vi "go_one_step.vi"(4 "执行完毕":bool, 5 "error in":errorcluster, 6 "Step":i32, 7 "Motor":i32, 8 "CmdLib In":refnum<k24>) -> (0 "error out":errorcluster, 1 "Position":i32, 2 "CmdLib Out":refnum<k24>)   [LabVIEW 2018]
uses:
  CmdLib.dll
  Verbal.vi
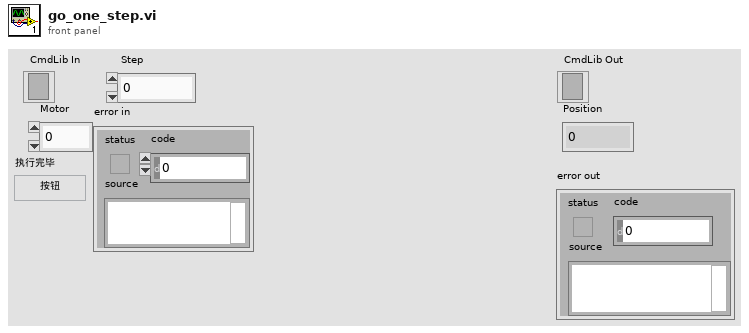
[diagram p1: front panel]
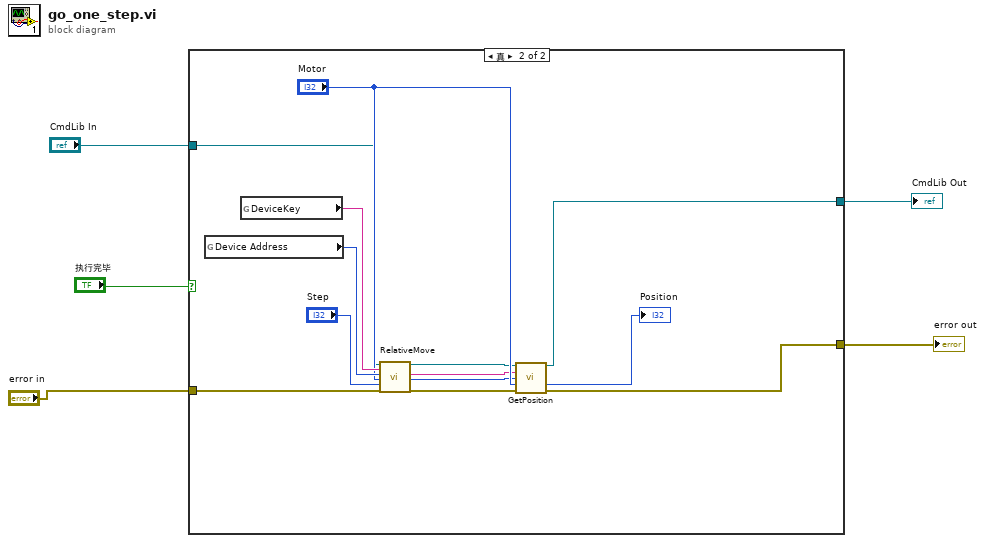
[diagram p0: block diagram]
diagram:
  n1 = case shown="真" "执行完毕" {
    tunnel: "CmdLib In" -> [w7 w11]
    tunnel: "error in" -> [w6 w10]
    tunnel: [w7 w9] -> w3
    tunnel: [w6 w8] -> w2
    frame False {
    }
    frame True {
      n2 = global read "Verbal.vi" "Device Address"() -> (w19:i32)
      n3 = global read "Verbal.vi" "DeviceKey"() -> (w20:string)
      n4 = call "RelativeMove.vi"("CmdLib In"=w11, "DeviceKey In"=w20, "Device Address In"=w19, "Motor"="Motor", "Relative Steps"="Step", "error in (no error)"=w10) -> ("CmdLib Out"=w15:refnum<k24>, "DeviceKey Out"=w14:string, "Device Address Out"=w13:i32, "error out"=w12:errorcluster)  [unwired: 10 in]
      n5 = call "GetPosition.vi"("CmdLib In"=w15, "DeviceKey In"=w14, "Device Address In"=w13, "Motor"="Motor", "error in (no error)"=w12) -> ("CmdLib Out"=w9:refnum<k24>, "Position"=→"Position":i32, "error out"=w8:errorcluster)  [unwired: 6 in, 2 out]
    }
  }
  "CmdLib Out" <- w3
  "error out" <- w2
